vi "_2_readcommandsfromexcel.vi"(1 "inout_chart":string[][](array[string])=[["H3C page5", "select channel 0", "select channel 0", "select channel 0", "select channel 0", "select channel 0", "select channel 0"], ["", "write 0 to 127", "modify byte 127", "modify byte 127", "modify byte 127", "modify byte 127", "modify byte 127"], ["", "", "write 128 to 255", "write 128 to 255", "modify byte 123 to 126", "write 128 to 255", ""], ["", "", "", "", "write 128 to 255", "", ""], ["ordinary", "", "", "", "", "", ""]], 2 "input_forindex":string="H3C page5") -> (0 "output":string[][](array[string]))   [LabVIEW 2011]
panel:
  out "子数组":string[](array[string])
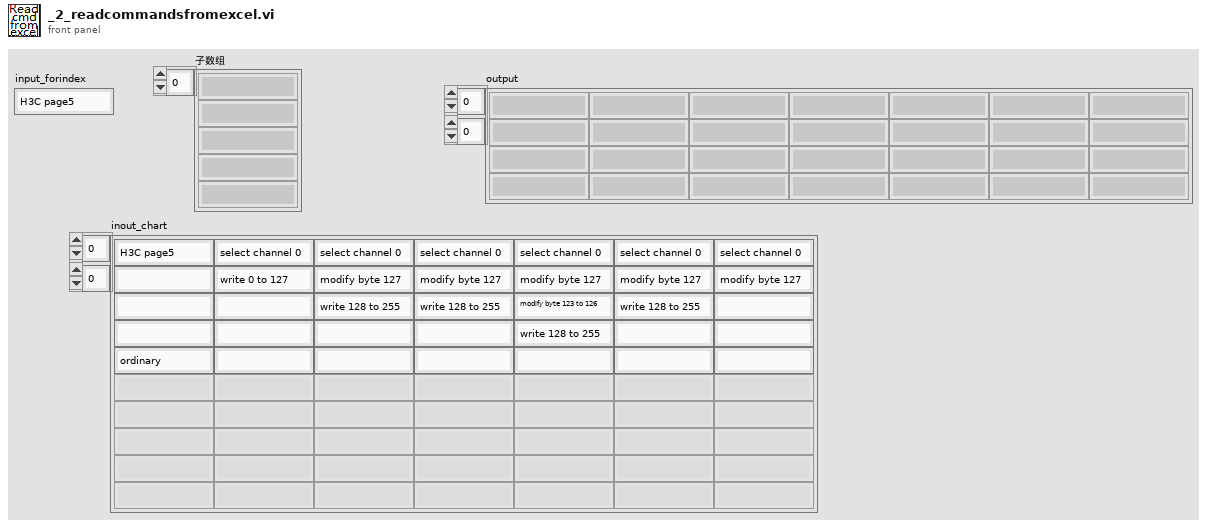
[diagram p1: front panel]
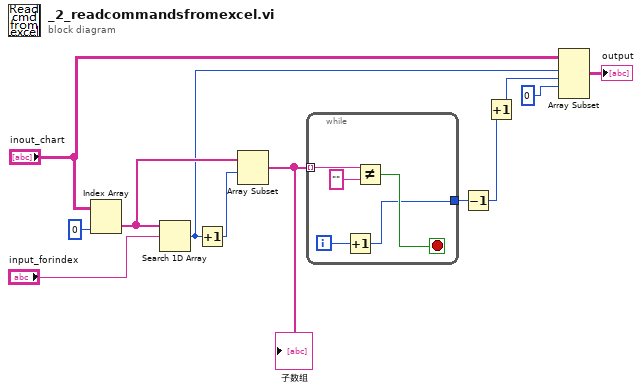
[diagram p0: block diagram]
diagram:
  n1 = Index Array(array="inout_chart", index (col)=0 ("禁用的索引 (列)")) -> (element=w10:string[])  [unwired: 1 in]
  n2 = Search 1D Array(1D array=w10, element="input_forindex") -> (index of element=w4:i32)  [unwired: 1 in]
  n3 = Increment(x=w4) -> (x+1=w8:i32)
  n4 = Array Subset(array=w10, index=w8) -> (w9:string[])  [unwired: 1 in]
  "子数组" <- w9
  n5 = while {
    tunnel: w9 -> [w17] mode=indexing
    tunnel: [w13] -> w7
    i -> [w14]
    stop <- w15 stop-if-true
    n6 = Increment(x=w14) -> (x+1=w13:i32)
    n7 = Not Equal?(x=w17, y="") -> (x != y?=w15:bool)
  }
  n8 = Decrement(x=w7) -> (x-1=w3:i32)
  n9 = Increment(x=w3) -> (x+1=w1:i32)
  n10 = Array Subset(array="inout_chart", index (row)=w4, length (row)=w1, index (col)=0 ("索引")) -> (→"output":string[][])  [unwired: 1 in]
